vi "heating.vi"(6 "T":u32[](array[numeric])=[1000, 10000, 300, 180000, 300, 5000, 180000, 3000], 7 "Alarm":bool[](array[boolean])=[FALSE, FALSE], 9 "ZB":bool[](array[boolean])=[FALSE, FALSE], 10 "XB":bool[](array[boolean])=[FALSE, FALSE, FALSE, FALSE, FALSE], 11 "Z_in":T5={"Z_HSw"=1, "Z_HSetState"=enum."on", "Z_ASetState"=enum."on", "Z_DSetState"=enum."on"}) -> (1 "ALR_ON":bool[](array[boolean]), 2 "YB":bool[](array[boolean]), 3 "Z":T1={"Z_Source"=enum."local disabled", "Z_SetState"=enum."on", "Z_State"=enum."alarm", "Z_State_T"=0, "ZM_State"=enum."initialization", "ZM_State_T"=0, "ALR  L1"=FALSE, "ALR  L2"=FALSE, "HH_run"=0}, 4 "ZM_State_next":u32)   [LabVIEW 2019, in "Heating.lvlib"]
uses:
  Heating.lvlib
  ctl/Z_State.ctl
  ctl/Z.ctl
  ctl/Y_source.ctl
  ctl/ZM_State.ctl
  Sequence/State1.vi
  Trigers/RS.vi
  Timer Delay/Timer.vi
panel:
  # "Alarm_L1"
  # "Alarm_L2"
  # "Ki_XB01 contactor on"
  # "Ki_XB02 contactor off"
  # "XB24 local hand on"
  # "heating end"
  # "cooling end"
  # "Ki_ZB01 contactor on reg"
  # "Ki_ZB02 contactor off reg"
  # "TsStop"
  # "T_check"
  # "T_start_delay"
  # "T_heat_start"
  # "T_stop_delay"
  # "T_set_min"
  # "T_heat_stop"
  # "T_restart_delay"
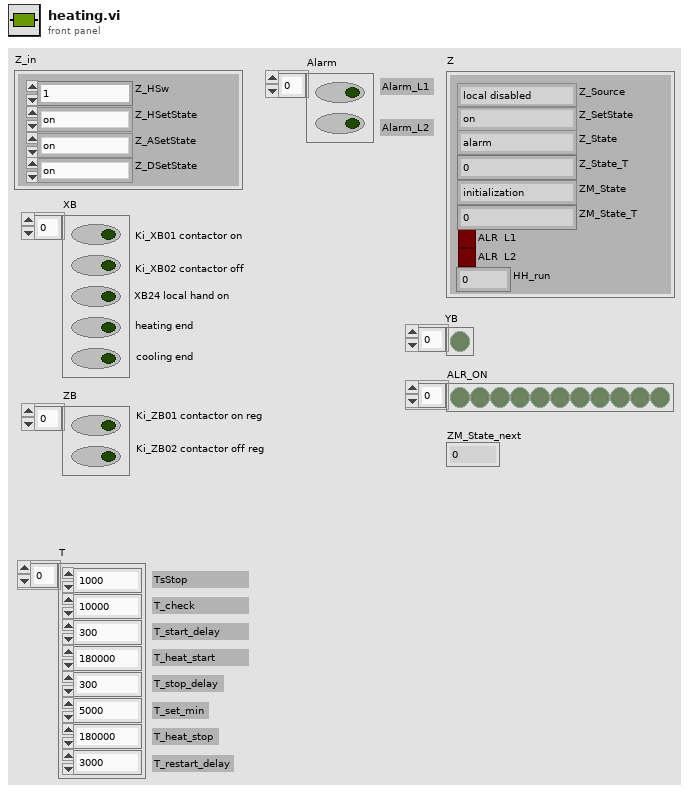
[diagram p1: front panel]
types:
  T1 = typedef "Heating.lvlib/Z.ctl" = cluster{"Z_Source":T2, "Z_SetState":T3, "Z_State":T3, "Z_State_T":u32, "ZM_State":T4, "ZM_State_T":u32, "ALR  L1":bool, "ALR  L2":bool, "HH_run":i32}
  T2 = typedef "Heating.lvlib/Y_source.ctl" = enum8{"initialize", "local disabled", "local hand", "hand", "auto", "dist"}
  T3 = typedef "Heating.lvlib/Z_State.ctl" = enum8{"initialization", "alarm", "disabled", "not ready", "stop ready", "reserv", "switched off", "reserv2", "switched on", "check", "on min", "decrease out", "on", "increase out", "on max"}
  T4 = typedef "Heating.lvlib/ZM_State.ctl" = enum8{"initialization", "stop", "start_cmd", "contactor_on_cmd", "heating", "on", "stop_cmd", "power_down", "contactor_off_cmd", "cooling", "restart_delay"}
  T5 = cluster{"Z_HSw":u32, "Z_HSetState":T3, "Z_ASetState":T3, "Z_DSetState":T3}
  T6 = cluster{"Z_Source":T2, "Z_SetState":T3, "ZM_State":T4}
  T7 = cluster{"Z_Source":T2, "Z_State":T3, "ZM_State":T4}
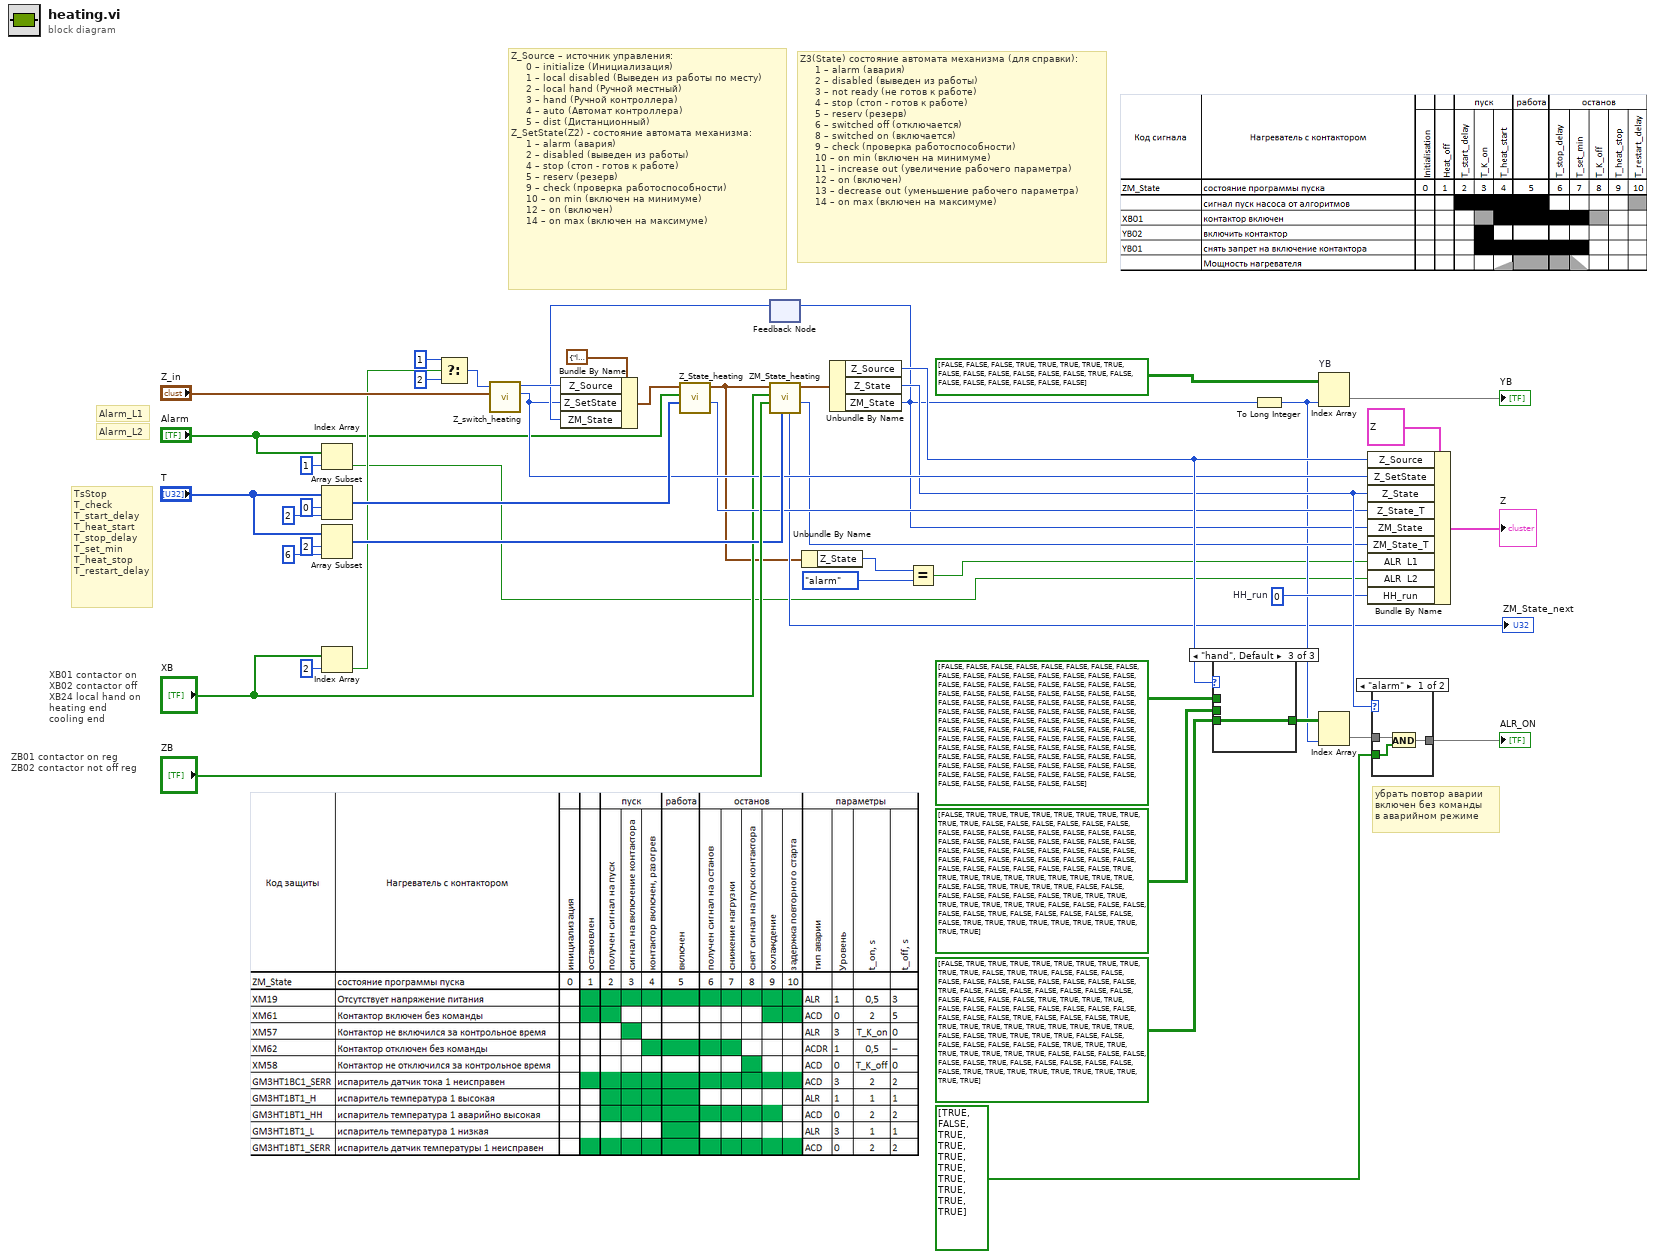
[diagram p0: block diagram]
diagram:
  w12 = 0  # HH_run
  # "Alarm_L2"
  # "Alarm_L1"
  # "ZB01 contactor on reg\nZB02 contactor not off reg"
  # "XB01 contactor on\nXB02 contactor off\nXB24 local hand on\nheating end\ncooling end"
  # "TsStop\nT_check\nT_start_delay\nT_heat_start\nT_stop_delay\nT_set_min\nT_heat_stop\nT_restart_delay"
  # "убрать повтор аварии\nвключен без команды\nв аварийном режиме"
  # "Z_Source – источник управления:\n     0 – initialize (Инициализация)\n     1 – local disabled (Выведен из работы по месту)\n     2 – local hand (Ручной местный)\n     3 – hand (Ручной контроллера)\n     4 – auto (Автомат контроллера)\n     5 – dist (Дистанционный)\nZ_SetState(Z2) - состояние автомата механизма:\n     1 – alarm (авария)\n     2 – disabled (выведен из работы)\n     4 – stop (стоп - готов к работе)\n     5 – reserv (резерв)\n     9 – check (проверка работоспособности)\n     10 – on min (включен на минимуме)\n     12 – on (включен)\n     14 – on max (включен на максимуме)"
  # "Z3(State) состояние автомата механизма (для справки):\n     1 – alarm (авария)\n     2 – disabled (выведен из работы)\n     3 – not ready (не готов к работе)\n     4 – stop (стоп - готов к работе)\n     5 – reserv (резерв)\n     6 – switched off (отключается)\n     8 – switched on (включается)\n     9 – check (проверка работоспособности)\n     10 – on min (включен на минимуме)\n     11 – increase out (увеличение рабочего параметра)\n     12 – on (включен)\n     13 – decrease out (уменьшение рабочего параметра)\n     14 – on max (включен на максимуме)"
  n1 = Index Array(array="Alarm", index=1) -> (element=w2:bool)
  n2 = Array Subset(array="T", index=0, length=2 ("index")) -> (w33:u32[])
  n3 = Array Subset(array="T", index=2, length=6 ("index")) -> (w37:u32[])
  n4 = Index Array(array="XB", index=2) -> (element=w22:bool)
  n5 = Select(t=u32 1, s=w22, f=u32 2) -> (s? t:f=w39:u32)
  n6 = call "Z_switch_heating.vi"("Z"="Z_in", "Z_LSw"=w39) -> ("Z_SetState"=w20:T3, "Z_Source"=w30:T2)  [unwired: 8 in]
  n7 = feedback #1() -> (w28:T4)  [unwired: 1 in]
  n8 = Bundle By Name(cluster=T6 {"Z_Source"=enum."local disabled", "Z_SetState"=enum."alarm", "ZM_State"=enum."initialization"} ("Z_In"), "Z_Source"=w30, "Z_SetState"=w20, "ZM_State"=w28) -> (w29:T6)
  n9 = call "Z_State_heating.vi"("Time"=w33, "Alarm"="Alarm", "Z_In"=w29) -> ("t"=w18:u32, "Z_Out"=w6:T7)  [unwired: 7 in]
  n10 = call "ZM_State_heating.vi"("T"=w37, "ZB"="ZB", "XB"="XB", "Z_In"=w6) -> ("t"=w16:u32, "Z_Out"=w32:T7, "ZM_State_next"=→"ZM_State_next":u32)  [unwired: 5 in]
  n11 = Unbundle By Name(w6) -> ("Z_State"=w5:T3)
  n12 = Unbundle By Name(w32) -> ("Z_Source"=w21:T2, "Z_State"=w19:T3, "ZM_State"=w17:T4)
  n13 = feedback-in #1(w17) -> ()
  n14 = Equal?(x=w5, y=Z_State."alarm") -> (x = y?=w4:bool)
  n15 = case shown="\"hand\", Default" w21 {
    tunnel: bool[][] [[FALSE, FALSE, FALSE, FALSE, FALSE, FALSE, FALSE, FALSE, FALSE, FALSE, FALSE], [FALSE, FALSE, FALSE, FALSE, FALSE, FALSE, FALSE, FALSE, FALSE, FALSE, FALSE], [FALSE, FALSE, FALSE, FALSE, FALSE, FALSE, FALSE, FALSE, FALSE, FALSE, FALSE], [FALSE, FALSE, FALSE, FALSE, FALSE, FALSE, FALSE, FALSE, FALSE, FALSE, FALSE], [FALSE, FALSE, FALSE, FALSE, FALSE, FALSE, FALSE, FALSE, FALSE, FALSE, FALSE], [FALSE, FALSE, FALSE, FALSE, FALSE, FALSE, FALSE, FALSE, FALSE, FALSE, FALSE], [FALSE, FALSE, FALSE, FALSE, FALSE, FALSE, FALSE, FALSE, FALSE, FALSE, FALSE], [FALSE, FALSE, FALSE, FALSE, FALSE, FALSE, FALSE, FALSE, FALSE, FALSE, FALSE], [FALSE, FALSE, FALSE, FALSE, FALSE, FALSE, FALSE, FALSE, FALSE, FALSE, FALSE], [FALSE, FALSE, FALSE, FALSE, FALSE, FALSE, FALSE, FALSE, FALSE, FALSE, FALSE]] -> [w48 _ _]
    tunnel: bool[][] [[FALSE, TRUE, TRUE, TRUE, TRUE, TRUE, TRUE, TRUE, TRUE, TRUE, TRUE], [FALSE, FALSE, FALSE, FALSE, FALSE, FALSE, FALSE, FALSE, FALSE, FALSE, FALSE], [FALSE, FALSE, FALSE, FALSE, FALSE, FALSE, FALSE, FALSE, FALSE, FALSE, FALSE], [FALSE, FALSE, FALSE, FALSE, FALSE, FALSE, FALSE, FALSE, FALSE, FALSE, FALSE], [FALSE, FALSE, FALSE, FALSE, FALSE, FALSE, FALSE, FALSE, FALSE, FALSE, FALSE], [FALSE, TRUE, TRUE, TRUE, TRUE, TRUE, TRUE, TRUE, TRUE, TRUE, TRUE], [FALSE, FALSE, TRUE, TRUE, TRUE, TRUE, FALSE, FALSE, FALSE, FALSE, FALSE], [FALSE, FALSE, TRUE, TRUE, TRUE, TRUE, TRUE, TRUE, TRUE, TRUE, FALSE], [FALSE, FALSE, FALSE, FALSE, FALSE, TRUE, FALSE, FALSE, FALSE, FALSE, FALSE], [FALSE, TRUE, TRUE, TRUE, TRUE, TRUE, TRUE, TRUE, TRUE, TRUE, TRUE]] -> [_ w49 _]
    tunnel: bool[][] [[FALSE, TRUE, TRUE, TRUE, TRUE, TRUE, TRUE, TRUE, TRUE, TRUE, TRUE], [FALSE, TRUE, TRUE, FALSE, FALSE, FALSE, FALSE, FALSE, FALSE, FALSE, FALSE], [FALSE, FALSE, FALSE, TRUE, FALSE, FALSE, FALSE, FALSE, FALSE, FALSE, FALSE], [FALSE, FALSE, FALSE, FALSE, TRUE, TRUE, TRUE, TRUE, FALSE, FALSE, FALSE], [FALSE, FALSE, FALSE, FALSE, FALSE, FALSE, FALSE, FALSE, TRUE, FALSE, FALSE], [FALSE, TRUE, TRUE, TRUE, TRUE, TRUE, TRUE, TRUE, TRUE, TRUE, TRUE], [FALSE, FALSE, TRUE, TRUE, TRUE, TRUE, FALSE, FALSE, FALSE, FALSE, FALSE], [FALSE, FALSE, TRUE, TRUE, TRUE, TRUE, TRUE, TRUE, TRUE, TRUE, FALSE], [FALSE, FALSE, FALSE, FALSE, FALSE, TRUE, FALSE, FALSE, FALSE, FALSE, FALSE], [FALSE, TRUE, TRUE, TRUE, TRUE, TRUE, TRUE, TRUE, TRUE, TRUE, TRUE]] -> [_ _ w50]
    tunnel: [w48 w49 w50] -> w45
    frame "local disabled" {
    }
    frame "local hand" {
    }
    frame "hand", Default {
    }
  }
  n16 = To Long Integer(number=w17) -> (32bit integer=w11:i32)
  n17 = Index Array "YB"(array=bool[][] [[FALSE, FALSE, FALSE, TRUE, TRUE, TRUE, TRUE, TRUE, FALSE, FALSE, FALSE], [FALSE, FALSE, FALSE, TRUE, FALSE, FALSE, FALSE, FALSE, FALSE, FALSE, FALSE]], index (col)=w11) -> (element=→"YB":bool[])  [unwired: 1 in]
  n18 = Index Array(array=w45, index (col)=w11) -> (element=w44:bool[])  [unwired: 1 in]
  n19 = Bundle By Name(cluster=T1 {"Z_Source"=enum."local disabled", "Z_SetState"=enum."on", "Z_State"=enum."alarm", "Z_State_T"=0, "ZM_State"=enum."initialization", "ZM_State_T"=0, "ALR  L1"=FALSE, "ALR  L2"=FALSE, "HH_run"=0} ("Z"), "Z_Source"=w21, "Z_SetState"=w20, "Z_State"=w19, "Z_State_T"=w18, "ZM_State"=w17, "ZM_State_T"=w16, "ALR  L1"=w4, "ALR  L2"=w2, "HH_run"=w12) -> (→"Z":T1)
  n20 = case shown="\"alarm\"" w19 {
    tunnel: bool[] [TRUE, FALSE, TRUE, TRUE, TRUE, TRUE, TRUE, TRUE, TRUE, TRUE] -> [w52 _]
    tunnel: w44 -> [w53 w54]
    tunnel: [w51 w54] -> w43
    frame "alarm" {
      n21 = And(x=w53, y=w52) -> (x .and. y?=w51:bool[])
    }
    frame "disabled", Default {
    }
  }
  "ALR_ON" <- w43
